vi "sub_check_and_autocreate_tag.vi"(6 "Tag Type Default Value":string, 7 "Tag Type Data Type":string(combo)="string", 8 "error in (no error)":errorcluster, 9 "Tag Type Key to create or update":string, 10 "Tag Type Label":string, 11 "daq.io type in in":T1={"daq.io ref"=refnum, "daq.io API Base"="", "Device Type Key"="", "Device Key"="", "Account ID"="", "online"=TRUE}) -> (0 "error out":errorcluster, 3 "daq.io type out":T1={"daq.io ref"=refnum, "daq.io API Base"="", "Device Type Key"="", "Device Key"="", "Account ID"="", "online"=TRUE})   [LabVIEW 2013, in "daqio minimal.lvlib"]
doc: "This VI autocreates a new Tag Type if required. \n- creates and adds a new Tag Type to the local device store\n- adds a Tag Type online"
uses:
  daqio minimal.lvlib
  _typedefs/daqio-Type.ctl
  <vilib>/httpClient/ClientHandle.ctl
  _typedefs/FGV_commands.ctl
  <vilib>/httpClient/LabVIEWHTTPClient.lvlib
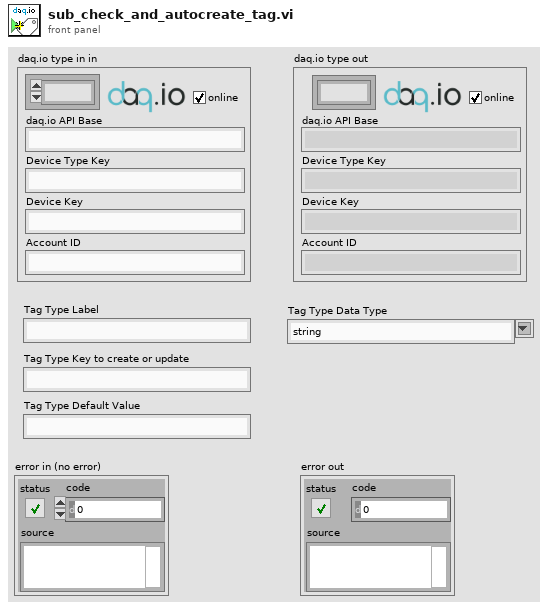
[diagram p1: front panel]
types:
  T1 = typedef "daqio minimal.lvlib/daqio-Type.ctl" = cluster{"daq.io ref":T2, "daq.io API Base":string, "Device Type Key":string, "Device Key":string, "Account ID":string, "online":bool}
  T2 = typedef "LabVIEWHTTPClient.lvlib/ClientHandle.ctl" = refnum<k1>
  T3 = typedef "daqio minimal.lvlib/FGV_commands.ctl" = enum16{"Init / update", "Edit Item", "Find or Add Item", "Remove Item", "Delete All"}
  T4 = typedef "daqio minimal.lvlib/daqio-Device-Type-Info-return.ctl" = cluster{"channel_types":T5[], "devices":T6[], "label":string, "event_types":T7[], "key":string, "tag_types":T8[], "id":string, "permissions":cluster{"write":string[], "read":string[]}}
  T5 = typedef "daqio minimal.lvlib/daqio-Channel-Type-POST-return.ctl" = cluster{"device_type_id":string, "id":string, "key":string, "label":string, "data_type":string, "permissions":cluster{"write":string[], "read":string[]}}
  T6 = typedef "daqio minimal.lvlib/daqio-Device.ctl" = cluster{"permissions":cluster{"write":string[], "read":string[]}, "id":string, "label":string, "key":string, "device_type_id":string, "tags":cluster{"key":string, "value":string}[], "files":string[]}
  T7 = typedef "daqio minimal.lvlib/daqio-Event-Type.ctl" = cluster{"device_type_id":string, "permissions":cluster{"read":string[], "write":string[]}, "id":string, "key":string, "label":string}
  T8 = typedef "daqio minimal.lvlib/daqio-Tag-Type-POST-return.ctl" = cluster{"label":string, "id":string, "device_type_id":string, "permissions":cluster{"write":string[], "read":string[]}, "default":string, "key":string}
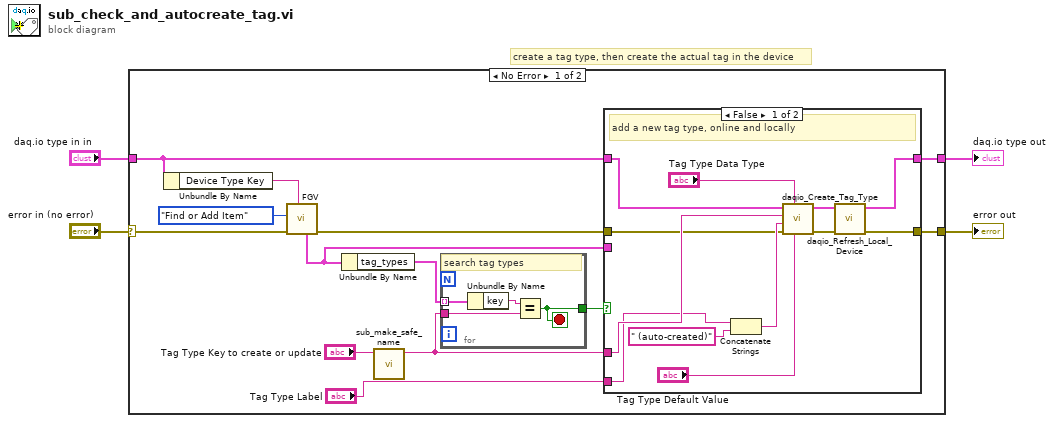
[diagram p0: block diagram]
diagram:
  # "create a tag type, then create the actual tag in the device"
  n1 = case shown="No Error" "error in (no error)" {
    selector: "error in (no error)" -> [w8 w37]
    tunnel: [w10 w37] -> w4
    tunnel: [w9 w36] -> w3
    tunnel: "daq.io type in in" -> [w7 w36]
    frame No Error {
      n2 = Unbundle By Name(w7) -> ("Device Type Key"=w6:string)
      n3 = call "FGV.vi"("Dev Type Key"=w6, "error in (no error)"=w8, "Action"=FGV_commands."Find or Add Item") -> ("error out"=w15:errorcluster, "Dev Type out"=w16:T4)  [unwired: 4 in, 3 out]
      n4 = Unbundle By Name(w16) -> ("tag_types"=w13:T8[])
      n5 = call "sub_make_safe_name.vi"("Input String"="Tag Type Key to create or update") -> ("Safe Output String"=w17:string)  [unwired: 10 in]
      n6 = for {
        tunnel: w13 -> [w35] mode=indexing
        tunnel: w17 -> [w33]
        tunnel: [w32] -> w14
        stop <- w32 stop-if-true
        # "search tag types"
        n7 = Unbundle By Name(w35) -> ("key"=w34:string)
        n8 = Equal?(x=w34, y=w33) -> (x = y?=w32:bool)
      }
      n9 = case shown="False" w14 {
        tunnel: w7 -> [w26 w31]
        tunnel: [w21 w31] -> w9
        tunnel: w17 -> [w27 _]
        tunnel: w15 -> [w22 w30]
        tunnel: [w23 w30] -> w10
        tunnel: w16 -> [_ _]
        tunnel: "Tag Type Label" -> [w20 _]
        frame False {
          # "add a new tag type, online and locally"
          n10 = Concatenate Strings(w20, " (auto-created)" ("string")) -> (w28:string)
          n11 = call "daqio_Create_Tag_Type.vi"("new Tag default value"="Tag Type Default Value", "new Tag  Data Type"="Tag Type Data Type", "error in (no error)"=w22, "new Tag Label"=w28, "new Tag Key"=w27, "daq.io type in"=w26) -> ("error out"=w24:errorcluster, "daq.io type out"=w25:T1)  [unwired: 2 in, 2 out]
          n12 = call "daqio_Refresh_Local_Device.vi"("error in (no error)"=w24, "daq.io type in"=w25) -> ("error out"=w23:errorcluster, "daq.io type out"=w21:T1)  [unwired: 5 in, 3 out]
        }
        frame True {
          # "don't add anything, it exists"
        }
      }
    }
    frame Error {
    }
  }
  "error out" <- w4
  "daq.io type out" <- w3
